vi "shuffle_taus.vi"(11 "Array In":dbl[](array[numeric])) -> (3 "Mixed Array Out":dbl[](array[numeric]))   [LabVIEW 2016]
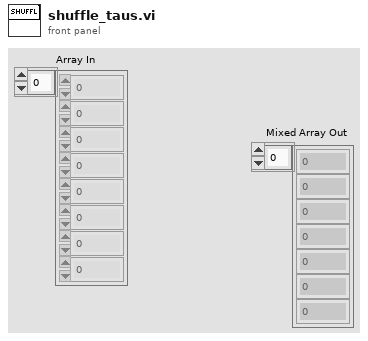
[diagram p1: front panel]
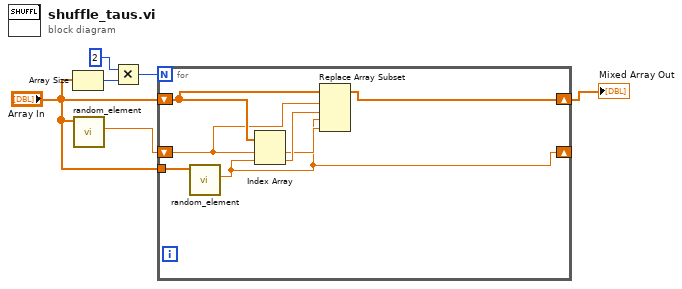
[diagram p0: block diagram]
diagram:
  n1 = Array Size(array="Array In") -> (size(s)=w2:i32)
  n2 = call "random_element.vi"("Array In"="Array In") -> ("Index"=w6:dbl)  [unwired: 9 in, 1 out]
  n3 = Multiply(x=2, y=w2) -> (x*y=w3:i32)
  n4 = for {
    N: w3 -> [_]
    shift-right: [w8] -> w5
    shift-left: "Array In" -> [w12]
    shift-right: [w7] -> _
    shift-left: w6 -> [w11]
    tunnel: "Array In" -> [w13]
    n5 = call "random_element.vi"("Array In"=w13) -> ("Index"=w7:dbl)  [unwired: 9 in, 1 out]
    n6 = Index Array(array=w12, index #1=w11, index #2=w7) -> (element #1=w9:dbl, element #2=w10:dbl)
    n7 = Replace Array Subset(array=w12, new element #1=w10, index #1=w11, new element #2=w9, index #2=w7) -> (w8:dbl[])
  }
  "Mixed Array Out" <- w5
